vi "pOGRAMA_POTENCIAS.vi"() -> ()   [LabVIEW 2013]
panel:
  out "Potencia":dbl
  out "Exponente":dbl
  out "Base":dbl
  # "GENERAR LA BASE Y EL EXPONENTE CON NUMEROS DE 1-10 \nLUEGO GENERAR LA POTENCIA USANDO EL CICLO FOR"
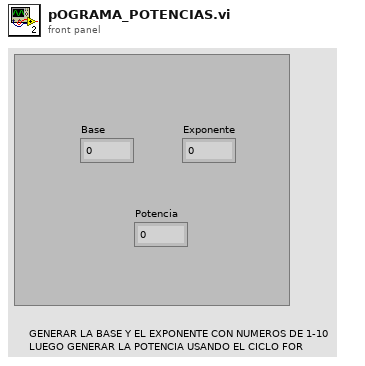
[diagram p1: front panel]
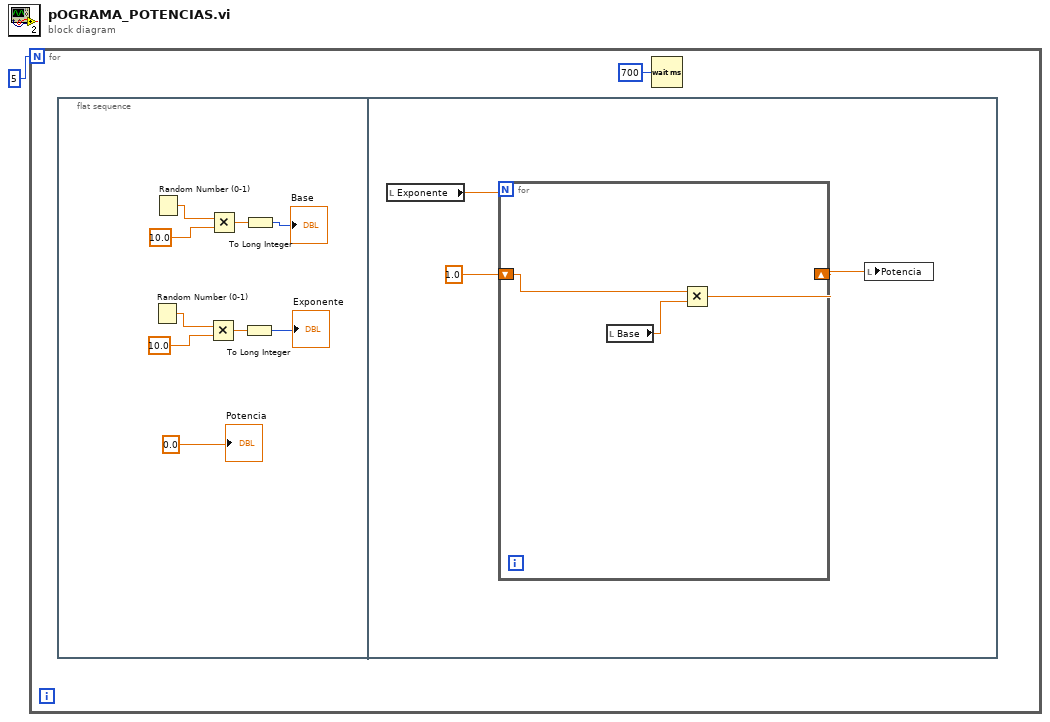
[diagram p0: block diagram]
diagram:
  n1 = for {
    N: 5 -> [_]
    n2 = flat-sequence {
      frame #0 {
        n3 = Random Number (0-1)() -> (number: 0 to 1=w5:dbl)
        n4 = Random Number (0-1)() -> (number: 0 to 1=w11:dbl)
        n5 = Multiply(x=w5, y=10.0) -> (x*y=w7:dbl)
        n6 = Multiply(x=w11, y=10.0) -> (x*y=w9:dbl)
        n7 = To Long Integer(number=w7) -> (32bit integer=→"Exponente":i32)
        n8 = To Long Integer(number=w9) -> (32bit integer=→"Base":i32)
        "Potencia" <- 0.0 ("Potencia")
      }
      frame #1 {
        n9 = local read "Exponente"() -> (w14:dbl)
        n10 = for {
          N: w14 -> [_]
          shift-right: [w15] -> w12
          shift-left: 1.0 ("y") -> [w17]
          n11 = local read "Base"() -> (w16:dbl)
          n12 = Multiply(x=w17, y=w16) -> (x*y=w15:dbl)
        }
        n13 = local write "Potencia"(w12) -> ()
      }
    }
    n14 = Wait (ms)(milliseconds to wait=u32 700) -> ()  [unwired: 1 out]
  }
